vi "Launch.vi"(10 "Actor":refnum<class "Actor.lvclass">, 11 "Helper Loop in":refnum<class "Helper Loop.lvclass">) -> (0 "error out":errorcluster, 1 "Dev Actor Refs":T1, 2 "Dev Actor Events":T2)   [LabVIEW 2021, in "Helper Loop.lvclass"]
uses:
  Helper Loop.lvclass
  <vilib>/jettl/jettl/Actor/Actor/Actor.lvclass
  Dev Actor Events.ctl
  Dev Actor Refs.ctl
  Event Loop Wrapper.vi
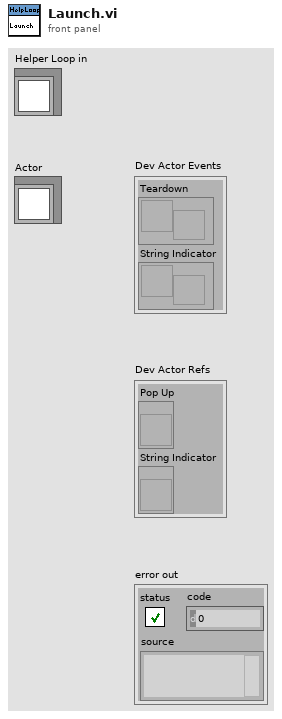
[diagram p1: front panel]
types:
  T1 = typedef "Dev Actor Refs.ctl" = cluster{"Pop Up":refnum<vi>, "String Indicator":refnum<vi>}
  T2 = typedef "Dev Actor Events.ctl" = cluster{"Teardown":refnum<user-event>, "String Indicator":refnum<user-event>}
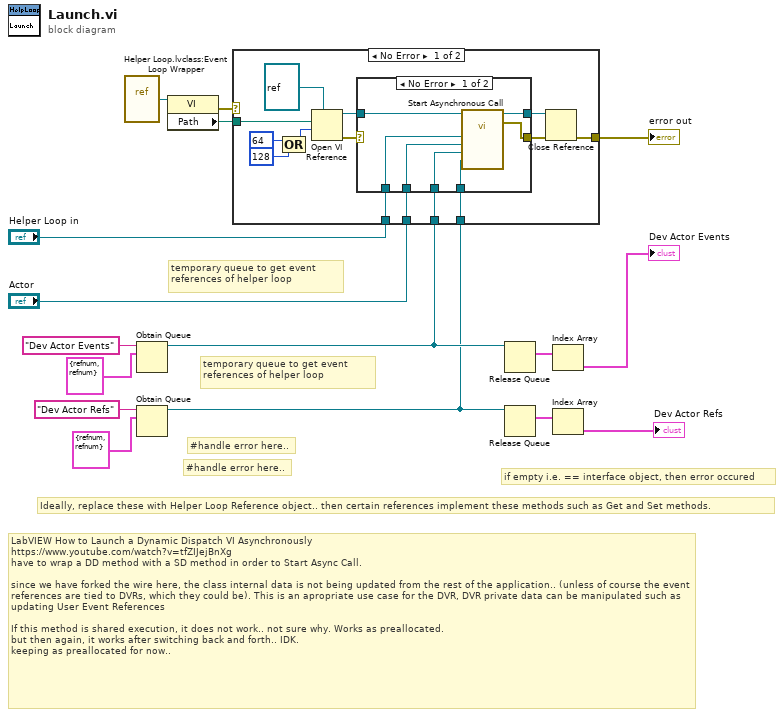
[diagram p0: block diagram]
diagram:
  # "temporary queue to get event references of helper loop"
  # "#handle error here.."
  # "#handle error here.."
  # "Ideally, replace these with Helper Loop Reference object.. then certain references implement these methods such as Get and Set methods."
  # "temporary queue to get event references of helper loop"
  # "if empty i.e. == interface object, then error occured"
  # "LabVIEW How to Launch a Dynamic Dispatch VI Asynchronously\nhttps://www.youtube.com/watch?v=tfZIJejBnXg\nhave to wrap a DD method with a SD method in order to Start Async Call.\n\nsince we have forked the wire here, the class internal data is not being updated from the rest of the application.. (unless of course the event references are tied to DVRs, which they could be). This is an apropriate use case for the DVR, DVR private data can be manipulated such as updating User Event References\n\nIf this method is shared execution, it does not work.. not sure why. Works as preallocated.\nbut then again, it works after switching back and forth.. IDK.\nkeeping as preallocated for now.."
  n1 = vi-ref "Helper Loop.lvclass:Event Loop Wrapper.vi"() -> (w12:refnum<vi>)
  n2 = Obtain Queue(name (unnamed)="Dev Actor Events", element data type=T2 {"Teardown"=refnum, "String Indicator"=refnum} ("Events")) -> (queue out=w8:refnum<queue>)  [unwired: 3 in, 2 out]
  n3 = Obtain Queue(name (unnamed)="Dev Actor Refs", element data type=T1 {"Pop Up"=refnum, "String Indicator"=refnum} ("Dev Actor Refs")) -> (queue out=w2:refnum<queue>)  [unwired: 3 in, 2 out]
  n4 = property class="VI"(reference=w12) -> (error out=w13:errorcluster, "Path"=w11:path)  [unwired: 1 in, 1 out]
  n5 = case shown="No Error" w13 {
    selector: w13 -> [_ w40]
    tunnel: [w28 w40] -> w16
    tunnel: w11 -> [w21 _]
    tunnel: "Actor" -> [w20 _]
    tunnel: "Helper Loop in" -> [w19 _]
    tunnel: w8 -> [w18 _]
    tunnel: w2 -> [w17 _]
    frame No Error {
      n6 = Compound Arithmetic op=OR(64 ("options: Multiple Clones,\n  Fire & Forget"), 128 ("options: Multiple Clones,\n  Fire & Forget")) -> (w26:i32)
      n7 = Open VI Reference(type specifier VI Refnum (for type only)=refnum<vi> refnum, vi path=w21, options=w26) -> (vi reference=w23:refnum<vi>, error out=w24:errorcluster)  [unwired: 3 in]
      n8 = case shown="No Error" w24 {
        selector: w24 -> [_ w39]
        tunnel: [w36 w38] -> w30
        tunnel: [w35 w39] -> w29
        tunnel: w23 -> [w37 w38]
        tunnel: w20 -> [w34 _]
        tunnel: w19 -> [w33 _]
        tunnel: w18 -> [w32 _]
        tunnel: w17 -> [w31 _]
        frame No Error {
          n9 = call-by-ref "Start Asynchronous Call"(reference=w37, "Dev Actor Refs"=w31, "Dev Actor Events"=w32, "Actor"=w34, "Helper Loop in"=w33) -> (reference out=w36:refnum<vi>, error out=w35:errorcluster)  [unwired: 9 in]
        }
        frame Error {
        }
      }
      n10 = Close Reference(reference=w30, error in (no error)=w29) -> (error out=w28:errorcluster)
    }
    frame Error {
    }
  }
  "error out" <- w16
  n11 = Release Queue(queue=w8) -> (remaining elements=w7:T2[])  [unwired: 2 in, 2 out]
  n12 = Release Queue(queue=w2) -> (remaining elements=w5:T1[])  [unwired: 2 in, 2 out]
  n13 = Index Array(array=w7) -> (element=→"Dev Actor Events":T2)  [unwired: 1 in]
  n14 = Index Array(array=w5) -> (element=→"Dev Actor Refs":T1)  [unwired: 1 in]
